vi "Handling AI param.vi"(4 "APCcode":i32[](array[numeric]), 5 "initialise":bool, 6 "AP":dbl[](array[numeric]), 7 "connect":bool[](array[boolean]), 8 "error in":errorcluster, 9 "input registers":u16[][](array[numeric]) format="%x", 10 "AIP":dbl[][](array[numeric]), 11 "AI in":T1) -> (0 "error":errorcluster, 3 "AI out":T1)   [LabVIEW 2019, in "Inputs.lvlib"]
uses:
  Inputs.lvlib
  Ctl/AI short.ctl
  Ctl/Parameter State.ctl
  Sensor limits calc.vi
  Sensor 2P.vi
  Filter/Filter_ext.vi
  Trigers/RS32_ext.vi
  Param limits calc.vi
  Sensor_limit_Hd.vi
  Sensor_limit_Ld.vi
  Sensor_limit_H.vi
  Sensor_limit_L.vi
  Timer Delay/Timers.lvlib
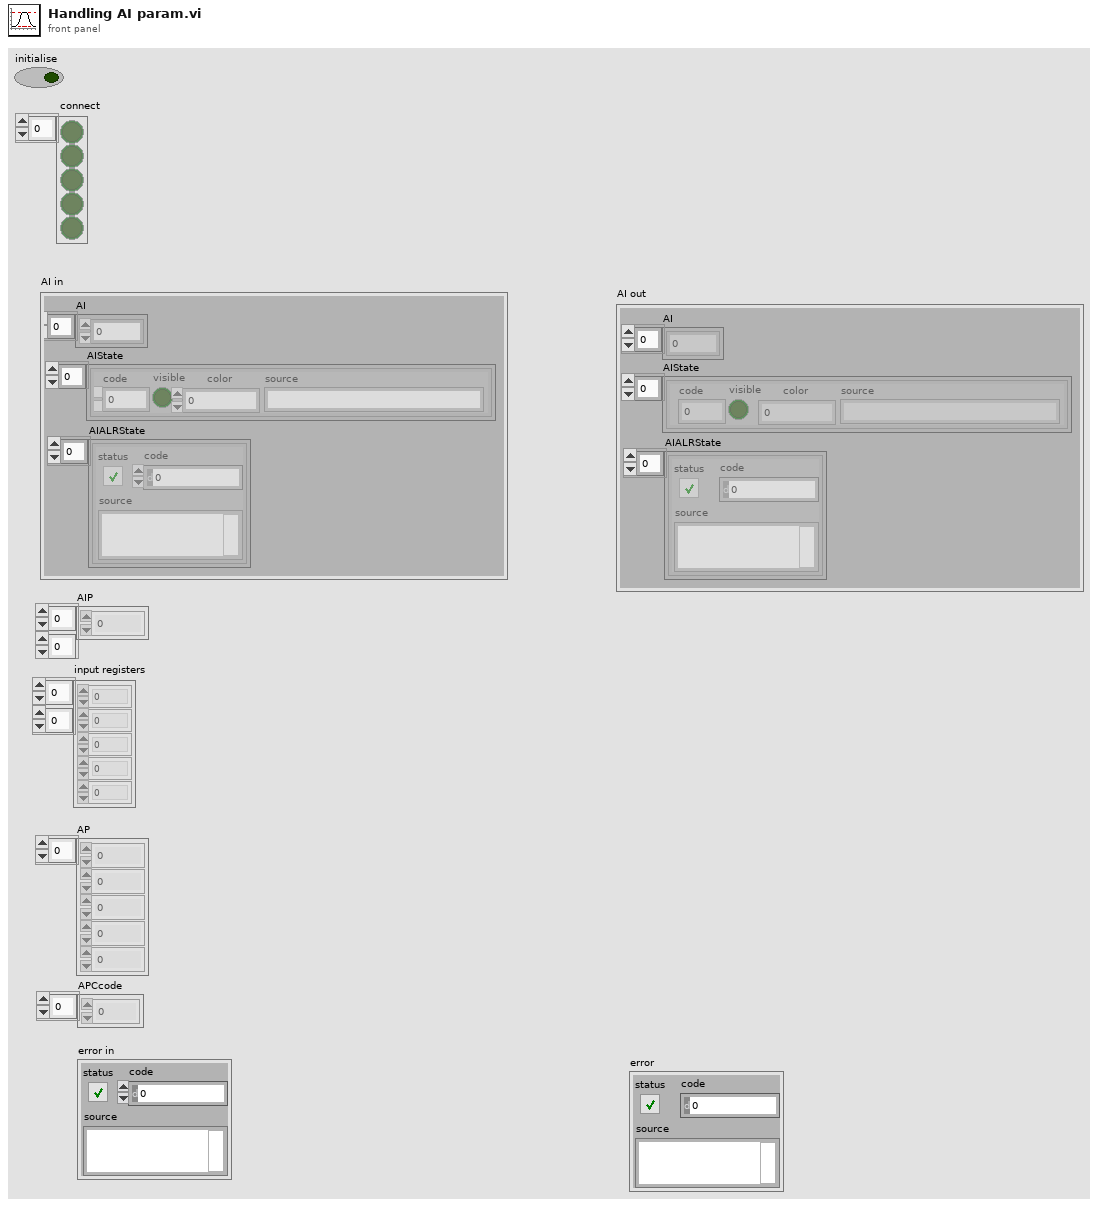
[diagram p1: front panel]
types:
  T1 = typedef "Inputs.lvlib/AI short.ctl" = cluster{"AI":dbl[], "AIState":T2[], "AIALRState":errorcluster[]}
  T2 = typedef "Inputs.lvlib/Parameter State.ctl" = cluster{"code":i32, "visible":bool, "color":u32, "source":string}
  T3 = cluster{"Filter PV_OUT":dbl, "Filter T":dbl, "Filter dT":dbl, "RS32 Q":u32}[]
  T4 = cluster{"Filter PV_OUT":dbl, "Filter T":dbl, "Filter dT":dbl, "RS32 Q":u32}
  T5 = cluster{"AIP[0]":dbl, "AIP[1]":dbl, "AIP[2]":dbl, "AIP[3]":dbl, "AIP[4]":dbl, "AIP[5]":dbl, "AIP[6]":dbl, "AIP[7]":dbl, "AIP[8]":dbl, "AIP[9]":dbl, "AIP[10]":dbl, "AIP[11]":dbl, "AIP[12]":dbl, "AIP[13]":dbl, "AIP[14]":dbl, "AIP[15]":dbl, "AIP[16]":dbl, "AIP[17]":dbl, "AIP[18]":dbl, "AIP[19]":dbl, "AIP[20]":dbl}
  T6 = cluster{"AIP[0]":dbl, "AIP[1]":dbl, "AIP[2]":dbl, "AIP[3]":dbl, "AIP[4]":dbl, "AIP[5]":dbl, "AIP[6]":dbl, "AIP[7]":dbl, "AIP[8]":dbl, "AIP[9]":dbl, "AIP[10]":dbl, "AIP[11]":dbl, "AIP[12]":dbl, "AIP[13]":dbl, "AIP[14]":dbl, "AIP[15]":dbl, "AIP[16]":dbl}
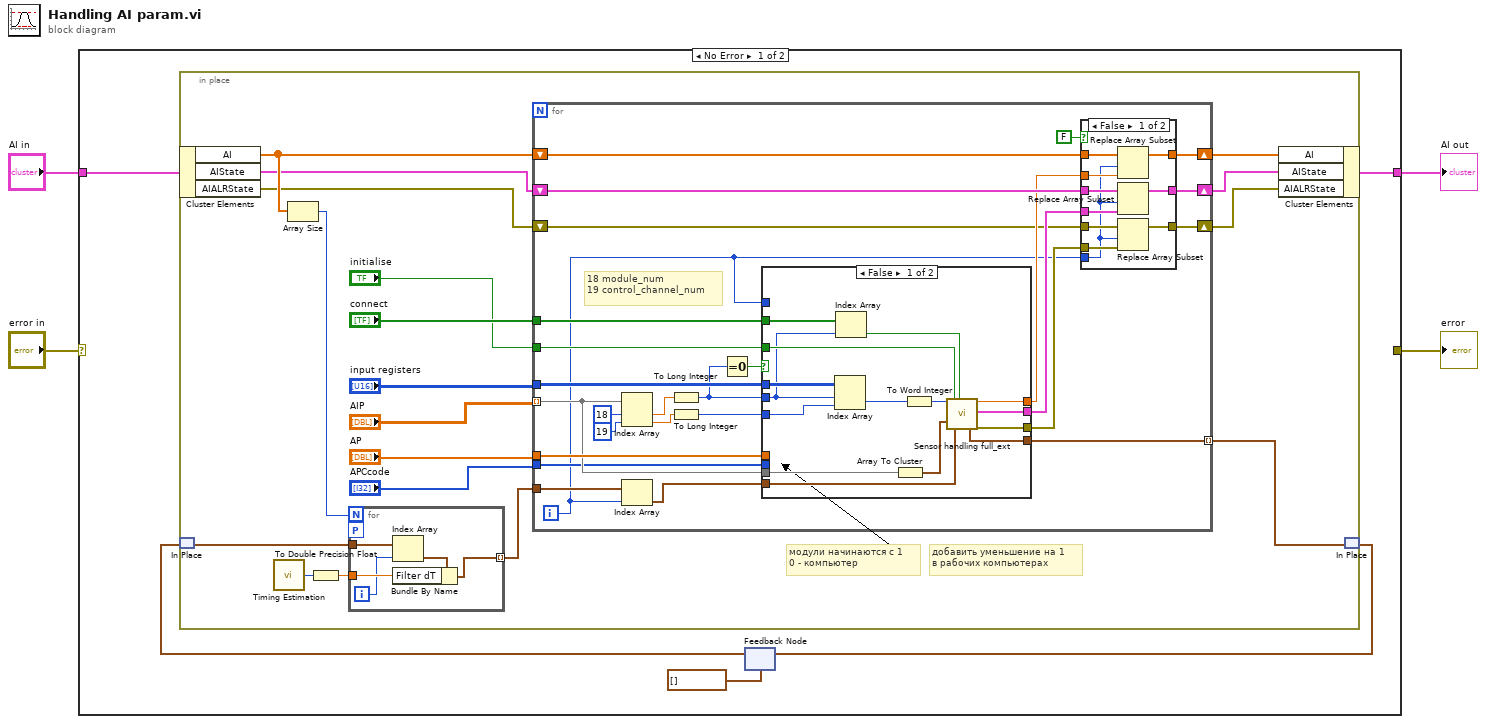
[diagram p0: block diagram]
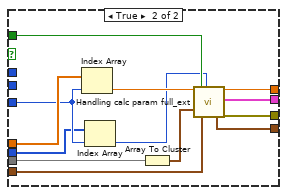
[diagram p2: hidden frame]
diagram:
  n1 = case shown="No Error" "error in" {
    selector: "error in" -> [_ w102]
    tunnel: [_ w102] -> w3
    tunnel: "AI in" -> [w8 w101]
    tunnel: [w7 w101] -> w1
    frame No Error {
      n2 = feedback #1(T3 []) -> (w6:T3)
      n3 = in-place {
        # "добавить уменьшение на 1\nв рабочих компьютерах"
        # "модули начинаются с 1\n0 - компьютер"
        n4 = in-place-cluster #2(w8) -> ("AI"=w18:dbl[], "AIState"=w17:T2[], "AIALRState"=w16:errorcluster[])
        n5 = in-place-match #3(w6) -> (w11:T3)
        n6 = call "Timing Estimation.vi"() -> ("dt (ms) out"=w23:u32)  [unwired: 9 in]
        n7 = Array Size(array=w18) -> (size(s)=w20:i32)
        n8 = To Double Precision Float(number=w23) -> (double precision float=w22:dbl)
        n9 = for {
          N: w20 -> [_]
          tunnel: w22 -> [w31]
          workers-P: _ -> [_]
          tunnel: w11 -> [w30]
          tunnel: [w32] -> w21 mode=indexing
          i -> [w28]
          n10 = Index Array(array=w30, index=w28) -> (element=w29:T4)
          n11 = Bundle By Name(cluster=w29, "Filter dT"=w31) -> (w32:T4)
        }
        n12 = for {
          tunnel: "AIP" -> [w43] mode=indexing
          tunnel: "input registers" -> [w56]
          tunnel: "connect" -> [w52]
          shift-right: [w53] -> w15
          shift-left: w18 -> [w55]
          shift-right: [w58] -> w14
          shift-left: w17 -> [w59]
          shift-right: [w49] -> w13
          shift-left: w16 -> [w48]
          tunnel: "initialise" -> [w47]
          tunnel: "AP" -> [w44]
          tunnel: "APCcode" -> [w42]
          tunnel: [w36] -> w10 mode=indexing
          tunnel: w21 -> [w35]
          i -> [w33]
          # "18 module_num\n19 control_channel_num"
          n13 = Index Array(array=w43, index #1=18 ("index (col)"), index #2=19 ("index (col)")) -> (element #1=w38:dbl, element #2=w37:dbl)
          n14 = Index Array(array=w35, index=w33) -> (element=w34:T4)
          n15 = To Long Integer(number=w38) -> (32bit integer=w45:i32)
          n16 = To Long Integer(number=w37) -> (32bit integer=w41:i32)
          n17 = Equal To 0?(x=w45) -> (x = 0?=w46:bool)
          n18 = case shown="False" w46 {
            tunnel: w43 -> [w74 w86]
            tunnel: [w73 w83] -> w57
            tunnel: w56 -> [w72 _]
            tunnel: [w70 w84] -> w54
            tunnel: w52 -> [w69 _]
            tunnel: w45 -> [w64 _]
            tunnel: w41 -> [w67 w81]
            tunnel: w47 -> [w66 w82]
            tunnel: w33 -> [_ _]
            tunnel: w44 -> [_ w87]
            tunnel: w42 -> [_ w80]
            tunnel: [w65 w78] -> w40
            tunnel: w34 -> [w61 w76]
            tunnel: [w60 w75] -> w36
            frame False {
              n19 = Index Array(array=w72, index (row)=w64, index (col)=w67) -> (element=w71:u16)
              n20 = Index Array(array=w69, index=w64) -> (element=w68:bool)
              n21 = Array To Cluster(array=w74) -> (cluster=w62:T5)
              n22 = To Word Integer(number=w71) -> (16bit integer=w63:i16)
              n23 = call "Sensor handling full_ext.vi"("PV"=w63, "control"=w62, "initialise"=w66, "Sensor handling full reg old"=w61, "connect"=w68) -> ("Sensor handling full reg"=w60:T4, "PVOUT"=w70:dbl, "STATE"=w73:T2, "ALRSTATE"=w65:errorcluster)  [unwired: 9 in, 2 out]
            }
            frame True {
              n24 = Index Array(array=w87, index=w81) -> (element=w85:dbl)
              n25 = Index Array(array=w80, index=w81) -> (element=w79:i32)
              n26 = Array To Cluster(array=w86) -> (cluster=w77:T6)
              n27 = call "Handling calc param full_ext.vi"("PV"=w85, "control"=w77, "initialise"=w82, "Sensor handling full reg old"=w76, "code"=w79) -> ("Sensor handling full reg"=w75:T4, "PVOUT"=w84:dbl, "STATE"=w83:T2, "ALRSTATE"=w78:errorcluster)  [unwired: 9 in, 2 out]
            }
          }
          n28 = case shown="False" FALSE {
            tunnel: w59 -> [w97 w99]
            tunnel: [w96 w99] -> w58
            tunnel: w57 -> [w95 _]
            tunnel: w55 -> [w94 w100]
            tunnel: w54 -> [w92 _]
            tunnel: [w93 w100] -> w53
            tunnel: w33 -> [w88 _]
            tunnel: w40 -> [w91 _]
            tunnel: w48 -> [w90 w98]
            tunnel: [w89 w98] -> w49
            frame False {
              n29 = Replace Array Subset(array=w94, new element=w92, index=w88) -> (w93:dbl[])
              n30 = Replace Array Subset(array=w97, new element=w95, index=w88) -> (w96:T2[])
              n31 = Replace Array Subset(array=w90, new element=w91, index=w88) -> (w89:errorcluster[])
            }
            frame True {
            }
          }
        }
        n32 = in-place-cluster #2("AI"=w15, "AIState"=w14, "AIALRState"=w13) -> (w7:T1)
        n33 = in-place-match #3(w10) -> (w5:T3)
      }
      n34 = feedback-in #1(w5) -> ()
    }
    frame Error {
    }
  }
  "error" <- w3
  "AI out" <- w1
